vi "ReadStdColour.vi"() -> ()   [LabVIEW 2017]
uses:
  <vilib>/MakerHub/LINX/Public/Utilities/Open Serial.vi
  <vilib>/MakerHub/LINX/LMH-LINX.lvlib
panel:
  out "数组":bool[](array[boolean])
  out "B coff":dbl format="%.6f"
  out "G coff":dbl format="%.6f"
  out "R coff":dbl format="%.6f"
  in  "CAL":bool
  out "Color":u32(colorbox) caption="颜色"
  out "Blue":u8
  out "Green":u8
  out "Red":u8
  in  "Next":bool
  # "标准色检测"
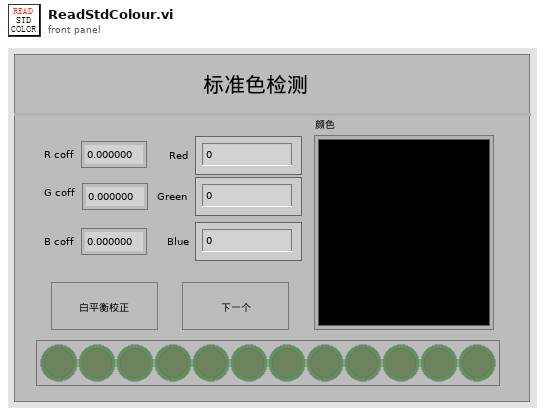
[diagram p1: front panel]
types:
  T1 = enum16{"open", "replace", "create", "open or create", "replace or create", "replace or create with confirmation"}
  T2 = typedef "LMH-LINX.lvlib/LINX Ref.ctl" = cluster{"IO":T3, "Interface":T4, "LINX Device Config":T5}
  T3 = typedef "LMH-LINX.lvlib/Platform.ctl" = enum16{"Remote", "Local"}
  T4 = typedef "LMH-LINX.lvlib/Interface.ctl" = enum16{"Serial", "TCP"}
  T5 = typedef "LMH-LINX.lvlib/Device.lvlib/LINX Device Config.ctl" = cluster{"Interface":T4, "COM Port":refnum<visa-resource-name>, "TCP Configuration":T6, "Device Family":u8, "Device ID":u8, "Device Name":string, "TCP Ref":refnum<k5>, "Channels":T7}
  T6 = typedef "LMH-LINX.lvlib/Device.lvlib/TCP Config.ctl" = cluster{"IP Address":string, "Port":u16}
  T7 = typedef "LMH-LINX.lvlib/Channels.ctl" = cluster{"DI":u8[], "DO":u8[], "AI":u8[], "AO":u8[], "PWM":u8[], "QE":u8[], "UART":u8[], "I2C 2":u8[], "SPI":u8[], "CAN":u8[], "Servo":u8[], "AI Ref (V)":dbl, "AI Resolution (Bits)":u8, "AO Ref (V)":dbl, "AO Resolution (Bits)":u8}
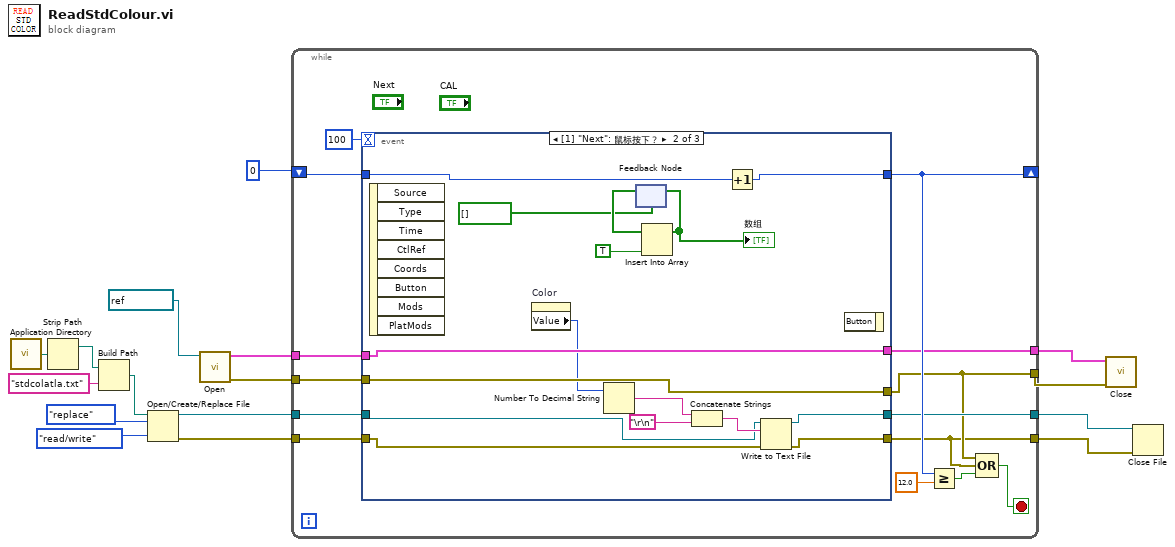
[diagram p0: block diagram]
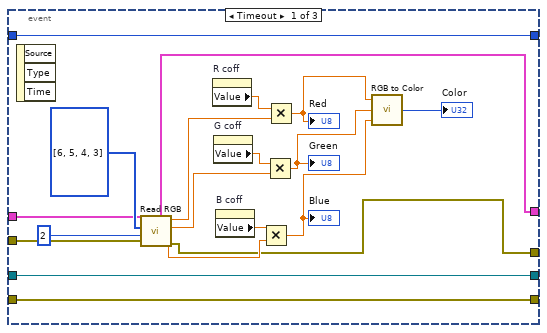
[diagram p2: hidden frame]
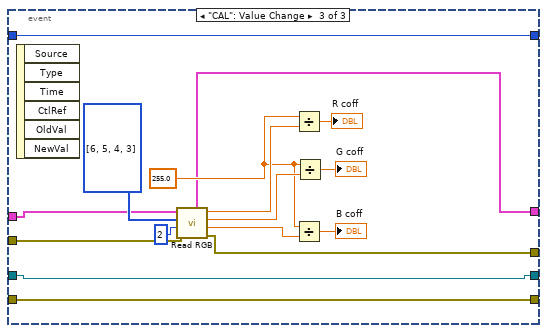
[diagram p3: hidden frame]
diagram:
  n1 = call <vilib>:"Application Directory.vi"() -> ("Application Directory"=w16:path)
  n2 = Strip Path(path=w16) -> (stripped path=w15:path)  [unwired: 1 out]
  n3 = Build Path(base path=w15, name or relative path="stdcolatla.txt" ("名称或相对路径")) -> (appended path=w11:path)
  n4 = Open/Create/Replace File(file path (use dialog)=w11, operation (0:open)=T1."replace" ("操作(0:open)"), access (0:read/write)=enum16{"read/write", "read-only", "write-only"}."read/write" ("权限(0:read/write)")) -> (refnum out=w8:refnum<file>, error out=w9:errorcluster)  [unwired: 3 in, 1 out]
  n5 = call-poly <vilib>:"Open.vi"("Serial Port"=refnum<visa-resource-name> "COM4") -> ("Error Out"=w4:errorcluster, "LINX Resource"=w5:T2)  [unwired: 8 in, 1 out]
  n6 = while {
    shift-right: [w28] -> _
    shift-left: 0 -> [w29]
    tunnel: w9 -> [w27]
    tunnel: w8 -> [w26]
    tunnel: [w19] -> w7
    tunnel: [w25] -> w6
    tunnel: w5 -> [w23]
    tunnel: w4 -> [w22]
    tunnel: [w21] -> w2
    tunnel: [w20] -> w1
    stop <- w17 stop-if-true
    n7 = event shown="[1] \"Next\": 鼠标按下？" {
      selector: _ -> [_ _ _]
      dyn-events: _ -> [_ _ _]
      timeout: 100 -> [_ _ _]
      tunnel: w29 -> [w34 w65 w74]
      tunnel: [w34 w64 w74] -> w28
      tunnel: w27 -> [w32 w55 w72]
      tunnel: w26 -> [w33 w54 w73]
      tunnel: [w32 w59 w72] -> w19
      tunnel: [w33 w60 w73] -> w25
      tunnel: w23 -> [w31 w58 w66]
      tunnel: w22 -> [w39 w57 w71]
      tunnel: [w35 w58 w70] -> w21
      tunnel: [w36 w57 w69] -> w20
      event Timeout {
        n8 = event-data() -> ()  [unwired: 1 in, 3 out]
        n9 = call "Read RGB.vi"("错误输入（无错误）"=w39, "Pulse OUT"=u8 2, "S0S1S2S3"=u8[] [6, 5, 4, 3] ("DO Channels"), "LINX Resource输入"=w31) -> ("错误输出"=w36:errorcluster, "Blue"=w47:dbl, "Green"=w48:dbl, "Red"=w49:dbl, "LINX Resource输出"=w35:T2)  [unwired: 3 in]
        n10 = property on="R coff" class="DigNum (严格)"() -> ("Value"=w43:dbl)  [unwired: 2 in, 2 out]
        n11 = property on="G coff" class="DigNum (严格)"() -> ("Value"=w42:dbl)  [unwired: 2 in, 2 out]
        n12 = property on="B coff" class="DigNum (严格)"() -> ("Value"=w41:dbl)  [unwired: 2 in, 2 out]
        n13 = Multiply(x=w41, y=w47) -> (x*y=w44:dbl)
        "Blue" <- w44
        n14 = Multiply(x=w42, y=w48) -> (x*y=w45:dbl)
        "Green" <- w45
        n15 = Multiply(x=w43, y=w49) -> (x*y=w46:dbl)
        "Red" <- w46
        n16 = call <vilib>:"RGB to Color.vi"("B"=w44, "G"=w45, "R"=w46) -> ("Color"=→"Color":u32)
      }
      event "Next": Mouse Down? {
        n17 = event-data() -> ()  [unwired: 1 in, 8 out]
        n18 = property on="Color" class="ColBox"() -> ("Value"=w56:u32)  [unwired: 2 in, 2 out]
        n19 = Number To Decimal String(number=w56) -> (decimal integer string=w63:string)  [unwired: 1 in]
        n20 = feedback #1(bool[] []) -> (w52:bool[])
        n21 = Insert Into Array(array=w52, new element=TRUE) -> (w50:bool[])  [unwired: 1 in]
        "数组" <- w50
        n22 = feedback-in #1(w50) -> ()
        n23 = Concatenate Strings(w63, "\r\n") -> (w61:string)
        n24 = Increment(x=w65) -> (x+1=w64:i32)
        n25 = Write to Text File(file (use dialog)=w54, text=w61, error in=w55) -> (refnum out=w60:refnum<file>, error out=w59:errorcluster)  [unwired: 1 in, 1 out]
        n26 = event-data() -> ()  [unwired: 2 in, 1 out]
      }
      event "CAL": Value Change {
        w78 = 255.0 ("x")
        n27 = event-data() -> ()  [unwired: 1 in, 6 out]
        n28 = call "Read RGB.vi"("错误输入（无错误）"=w71, "Pulse OUT"=u8 2, "S0S1S2S3"=u8[] [6, 5, 4, 3] ("DO Channels"), "LINX Resource输入"=w66) -> ("错误输出"=w69:errorcluster, "Blue"=w79:dbl, "Green"=w80:dbl, "Red"=w81:dbl, "LINX Resource输出"=w70:T2)  [unwired: 3 in]
        n29 = Divide(x=w78, y=w81) -> (x/y=→"R coff":dbl)
        n30 = Divide(x=w78, y=w79) -> (x/y=→"B coff":dbl)
        n31 = Divide(x=w78, y=w80) -> (x/y=→"G coff":dbl)
      }
    }
    n32 = Greater Or Equal?(x=w28, y=12.0) -> (x >= y?=w18:bool)
    n33 = Compound Arithmetic op=OR ("复合运算")(w20, w19, w18) -> (w17:bool)
  }
  n34 = call <vilib>:"Close.vi"("Error In"=w1, "LINX Resource"=w2) -> ()  [unwired: 9 in, 1 out]
  n35 = Close File(refnum=w6, error in=w7) -> ()  [unwired: 2 out]
